vi "_iWorx - Microphone.vi"() -> ()   [LabVIEW 2012]
uses:
  <vilib>/DAQmx/create/channels.llb/DAQmx Create Channel (AI-Voltage-Basic).vi
  <vilib>/DAQmx/configure/timing.llb/DAQmx Timing (Sample Clock).vi
  <vilib>/DAQmx/read.llb/DAQmx Read (Analog 1D Wfm NChan NSamp).vi
panel:
  in  "Reset Scale":bool
  in  "Log Info Button":bool
  in  "Set Up":bool
  in  "Channel":enum16{"Right", "Left", "Both"}(ring)
  in  "Pause Button":bool
  in  "Snapshot":bool
  in  "Stop":bool
  out "Waveform Chart":waveform(dbl)[](graph)
  in  "Clear Chart":bool
  in  "Open Log":bool
  in  "Rescale Y":bool
  # "iWorx - Microphone - Data Logger"
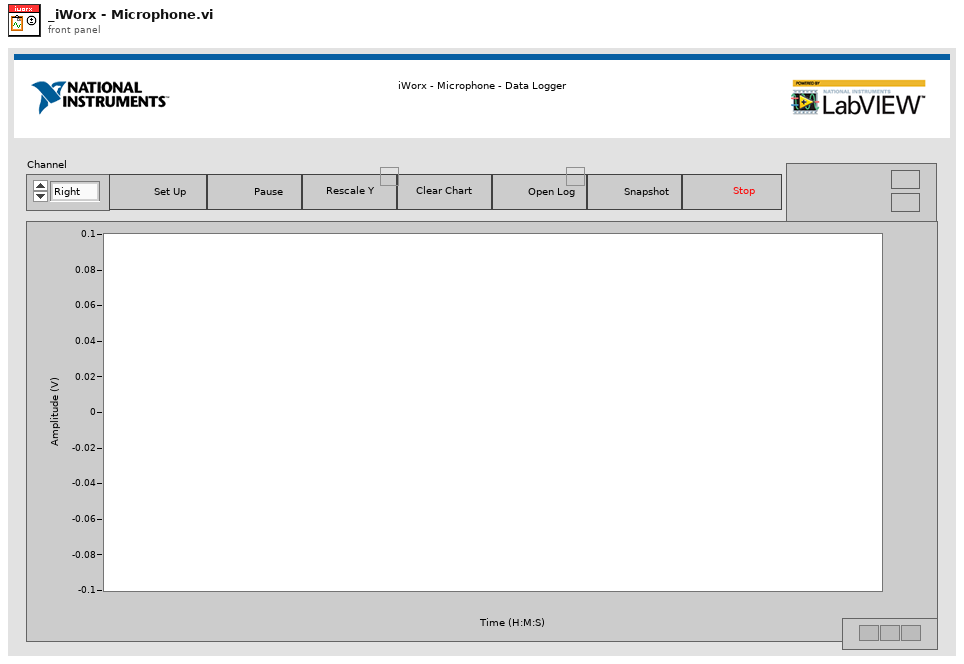
[diagram p1: front panel]
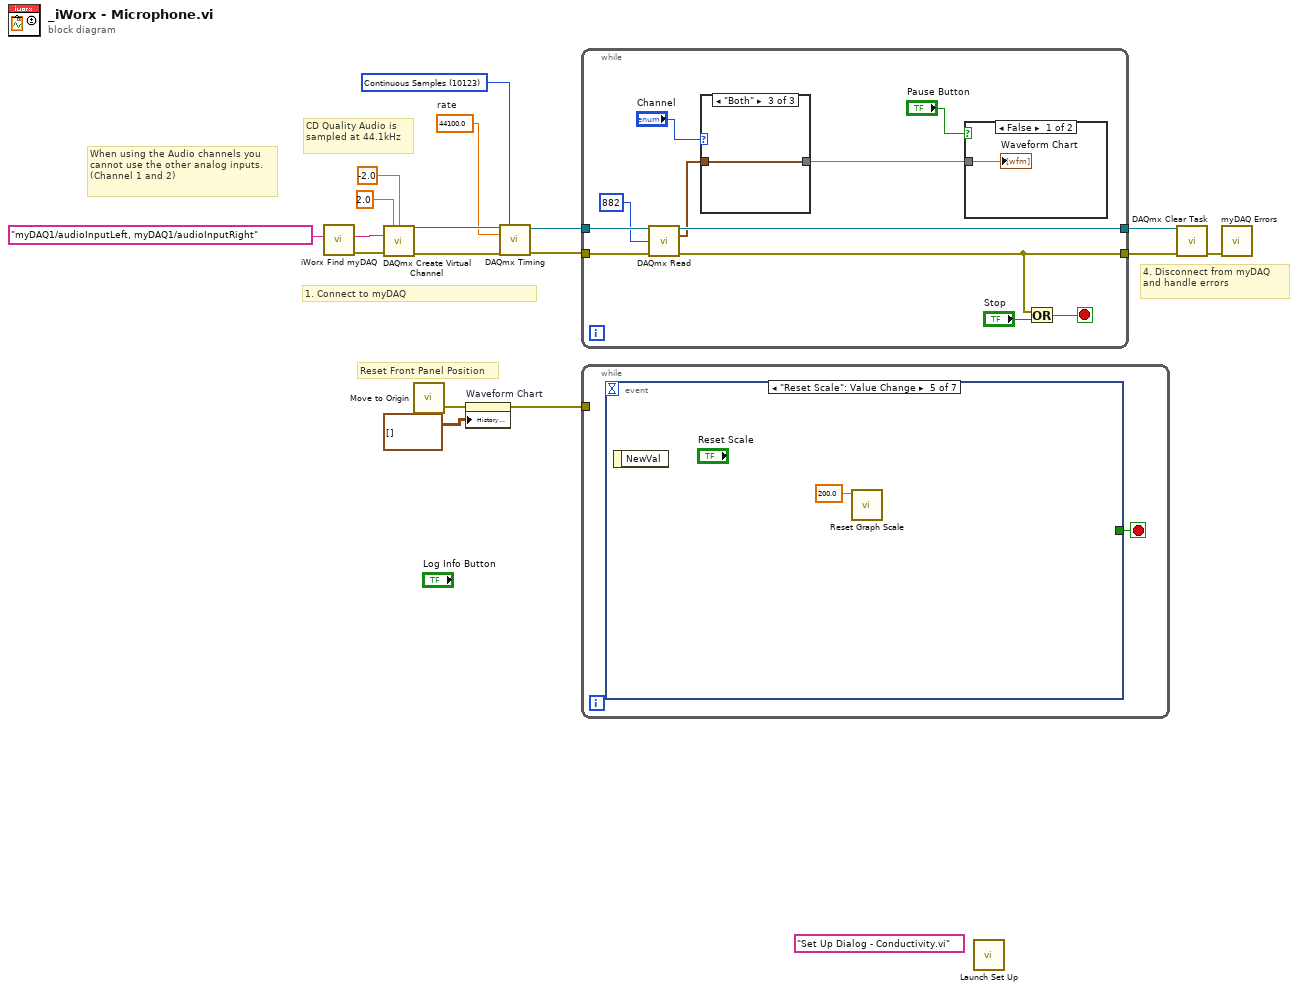
[diagram p0: block diagram]
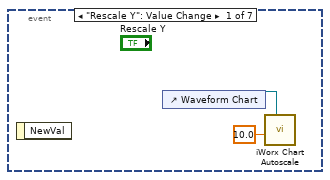
[diagram p2: hidden frame]
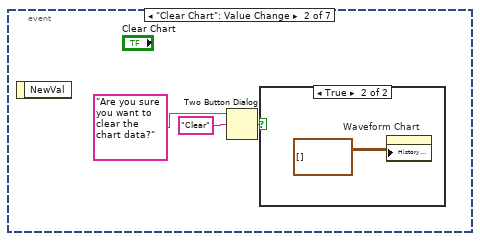
[diagram p3: hidden frame]
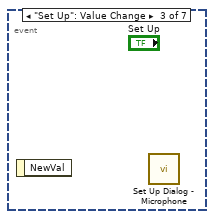
[diagram p5: hidden frame]
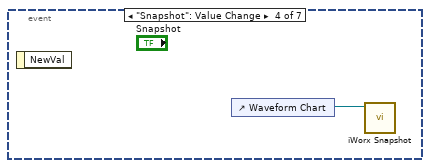
[diagram p6: hidden frame]
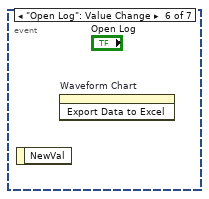
[diagram p7: hidden frame]
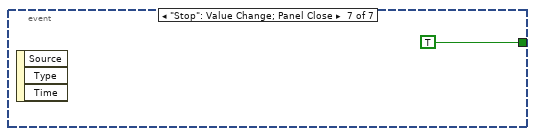
[diagram p8: hidden frame]
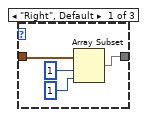
[diagram p9: hidden frame]
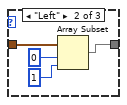
[diagram p10: hidden frame]
diagram:
  (unwired) "Set Up Dialog - Conductivity.vi" ("name or relative path")
  w9 = 44100.0  # rate
  w10 = 10123 items=["Finite Samples"=10178, "Continuous Samples"=10123, "Hardware Timed Single Point"=12522] ("sample mode")
  # "Reset Front Panel Position"
  # "4. Disconnect from myDAQ and handle errors"
  # "1. Connect to myDAQ"
  # "When using the Audio channels you cannot use the other analog inputs. (Channel 1 and 2)"
  # "CD Quality Audio is sampled at 44.1kHz"
  n1 = call "iWorx Find myDAQ.vi"("Preferred myDAQ (myDAQ1)"=tag "myDAQ1/audioInputLeft, myDAQ1/audioInputRight" ("physical channels")) -> ("Error Out"=w3:errorcluster, "DAQmx Physical Channel"=w2:tag)  [unwired: 6 in, 3 out]
  n2 = call-poly <vilib>:"DAQmx Create Virtual Channel.vi"("maximum value"=2.0, "minimum value"=-2.0, "physical channels"=w2, "error in"=w3) -> ("task out"=w14:refnum<k21>, "error out"=w13:errorcluster)  [unwired: 10 in]
  n3 = call "Move to Origin.vi"() -> ("Error Out"=w5:errorcluster)  [unwired: 3 in]
  n4 = property on="Waveform Chart" class="WFChart (strict)"(error in=w5, "History Data"=waveform(dbl)[][] []) -> (error out=w15:errorcluster)  [unwired: 1 in, 1 out]
  n5 = call-poly <vilib>:"DAQmx Timing.vi"("task/channels in"=w14, "sample mode"=w10, "rate"=w9, "error in"=w13) -> ("task out"=w11:refnum<k21>, "error out"=w12:errorcluster)  [unwired: 10 in]
  n6 = while {
    tunnel: w11 -> [w27]
    tunnel: [w26] -> w17
    tunnel: w12 -> [w25]
    tunnel: [w23] -> w16
    stop <- w24 stop-if-true
    n7 = call-poly <vilib>:"DAQmx Read.vi"("task/channels in"=w27, "number of samples per channel"=882 ("samples per channel"), "error in"=w25) -> ("task out"=w26:refnum<k21>, "data"=w20:waveform(dbl)[], "error out"=w23:errorcluster)  [unwired: 10 in]
    n8 = case shown="\"Both\"" "Channel" {
      tunnel: w20 -> [w30 w36 w37]
      tunnel: [w29 w35 w37] -> w18
      frame "Right", Default {
        n9 = Array Subset(array=w30, index=1, length=1) -> (w29:waveform(dbl)[])
      }
      frame "Left" {
        n10 = Array Subset(array=w36, index=0, length=1) -> (w35:waveform(dbl)[])
      }
      frame "Both" {
      }
    }
    n11 = case shown="False" "Pause Button" {
      tunnel: w18 -> [w38 _]
      frame False {
        "Waveform Chart" <- w38
      }
      frame True {
      }
    }
    n12 = Or(x=w23, y="Stop") -> (x .or. y?=w24:bool)
  }
  n13 = while {
    tunnel: w15 -> [_]
    stop <- w39 stop-if-true
    n14 = event shown="[4] \"Reset Scale\": Value Change" {
      selector: _ -> [_ _ _ _ _ _ _]
      dyn-events: _ -> [_ _ _ _ _ _ _]
      timeout: _ -> [_ _ _ _ _ _ _]
      tunnel: [_ _ _ _ _ _ TRUE] -> w39
      event "Rescale Y": Value Change {
        n15 = event-data() -> ()  [unwired: 1 in, 1 out]
        n16 = control-ref of="Waveform Chart"() -> (w40:refnum<vi>)
        n17 = call "iWorx Chart Autoscale.vi"("Selection Chart"=w40, "Rounding Multiple (1)"=10.0) -> ()  [unwired: 7 in, 3 out]
      }
      event "Clear Chart": Value Change {
        n18 = event-data() -> ()  [unwired: 1 in, 1 out]
        n19 = Two Button Dialog(message="Are you sure you want to clear the chart data?", 2:"Clear" ("T button name (\"OK\")")) -> (T button?=w43:bool)  [unwired: 1 in]
        n20 = case shown="True" w43 {
          frame False {
          }
          frame True {
            n21 = property on="Waveform Chart" class="WFChart (strict)"("History Data"=waveform(dbl)[][] []) -> ()  [unwired: 2 in, 2 out]
          }
        }
      }
      event "Set Up": Value Change {
        n22 = event-data() -> ()  [unwired: 1 in, 1 out]
        n23 = call "Set Up Dialog - Microphone.vi"() -> ()  [unwired: 12 in]
      }
      event "Snapshot": Value Change {
        n24 = event-data() -> ()  [unwired: 1 in, 1 out]
        n25 = control-ref of="Waveform Chart"() -> (w46:refnum<vi>)
        n26 = call "iWorx Snapshot.vi"("WaveformChart in"=w46) -> ()  [unwired: 10 in, 1 out]
      }
      event "Reset Scale": Value Change {
        n27 = event-data() -> ()  [unwired: 1 in, 1 out]
        n28 = call "Reset Graph Scale.vi"("Maximum (100)"=200.0) -> ()  [unwired: 11 in]
      }
      event "Open Log": Value Change {
        n29 = event-data() -> ()  [unwired: 1 in, 1 out]
        n30 = invoke on="Waveform Chart" class="WFChart (strict)" method="Export Data to Excel"() -> ()  [unwired: 3 in, 3 out]
      }
      event "Stop": Value Change; Panel Close {
        n31 = event-data() -> ()  [unwired: 1 in, 3 out]
      }
    }
  }
  n32 = call "Launch Set Up.vi"() -> ()  [unwired: 10 in, 2 out]
  n33 = call <vilib>:"DAQmx Clear Task.vi"("task in"=w17, "error in"=w16) -> ("error out"=w1:errorcluster)  [unwired: 13 in]
  n34 = call "myDAQ Errors.vi"("error in (no error)"=w1) -> ()  [unwired: 10 in, 1 out]
